vi "next chunk -- action stack.vi"(7 "stack action":T2, 8 "action list in":T1[](array[typedef]), 9 "next chunk action":T1=enum."init - uniform", 11 "command stack":T1[](array[typedef])) -> (1 "next chunk action out":T1=enum."init - uniform", 2 "stack is empty ?":bool, 3 "command stack out":T1[](array[typedef]))   [LabVIEW 2015]
uses:
  stack action -- control.ctl
  next chunk -- action.ctl
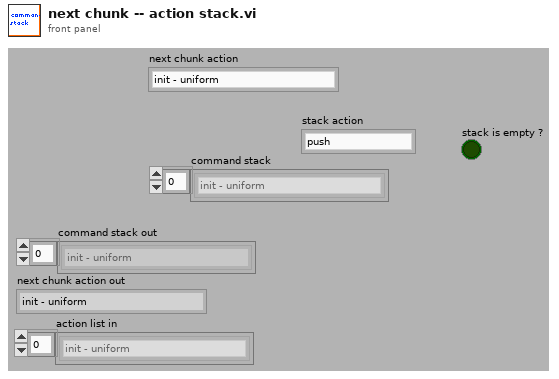
[diagram p1: front panel]
types:
  T1 = typedef "next chunk -- action.ctl" = enum16{"empty", "init - uniform", "next chunk - uniform", "next chunk - peaks are known", "init - peaks are known", ""}
  T2 = typedef "stack action -- control.ctl" = enum16{"push", "pop", "check", "init"}
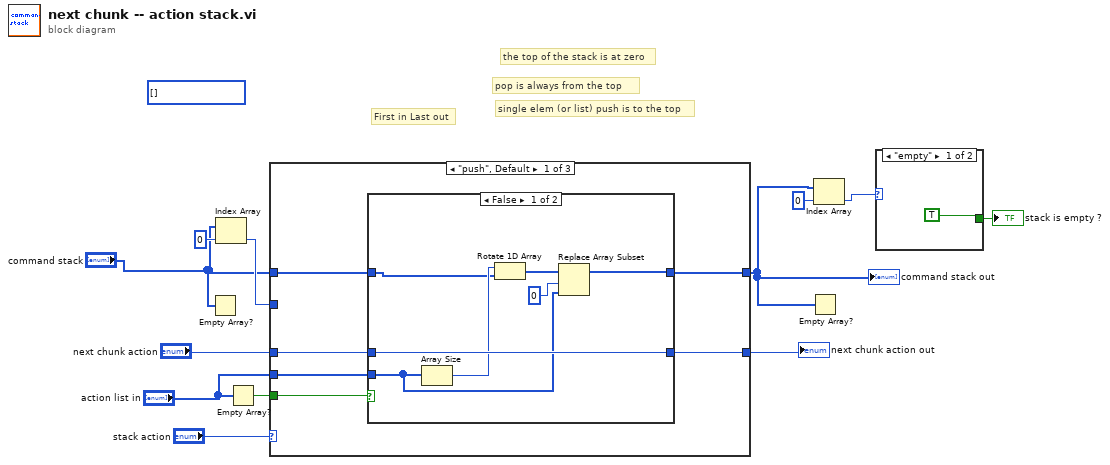
[diagram p0: block diagram]
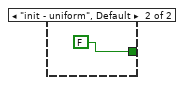
[diagram p2: hidden frame]
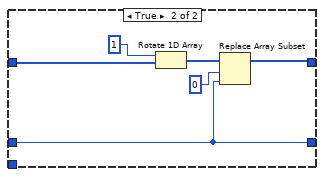
[diagram p3: hidden frame]
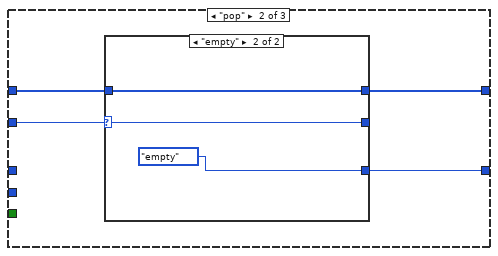
[diagram p4: hidden frame]
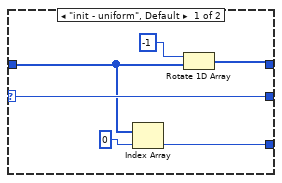
[diagram p5: hidden frame]
diagram:
  (unwired) T1[] [] items=["empty", "init - uniform", "next chunk - uniform", "next chunk - peaks are known", "init - peaks are known", ""] ("command stack")
  # "single elem (or list) push is to the top"
  # "pop is always from the top"
  # "First in Last out"
  # "the top of the stack is at zero"
  n1 = Empty Array?(array="command stack") -> ()  [unwired: 1 out]
  n2 = Index Array(array="command stack", index=0) -> (element=w9:T1)
  n3 = Empty Array?(array="action list in") -> (empty?=w11:bool)
  n4 = case shown="\"push\", Default" "stack action" {
    tunnel: [w18 w35 w45] -> w2
    tunnel: "command stack" -> [w17 w34 w45]
    tunnel: w9 -> [_ w33 _]
    tunnel: [w13 w32 w46] -> w3
    tunnel: "next chunk action" -> [w16 _ w46]
    tunnel: w11 -> [w15 _ _]
    tunnel: "action list in" -> [w14 _ _]
    frame "push", Default {
      n5 = case shown="False" w15 {
        tunnel: [w19 w26] -> w18
        tunnel: w17 -> [w23 w28]
        tunnel: w16 -> [w25 w29]
        tunnel: w14 -> [w20 _]
        tunnel: [w25 w29] -> w13
        frame False {
          n6 = Array Size(array=w20) -> (size(s)=w24:i32)
          n7 = Rotate 1D Array(1:w23, 2:w24) -> (0:w22:T1[])
          n8 = Replace Array Subset(array=w22, new element=w20, index=0) -> (w19:T1[])
        }
        frame True {
          n9 = Rotate 1D Array(1:w28, 2:1) -> (0:w31:T1[])
          n10 = Replace Array Subset(array=w31, new element=w29, index=0) -> (w26:T1[])
        }
      }
    }
    frame "pop" {
      n11 = case shown="\"empty\"" w33 {
        selector: w33 -> [w39 w43]
        tunnel: [w38 w44] -> w35
        tunnel: w34 -> [w36 w44]
        tunnel: [w40 next_chunk_--_action."empty" ("next chunk action")] -> w32
        tunnel: [w39 w43] -> _
        frame "init - uniform", Default {
          n12 = Index Array(array=w36, index=0) -> (element=w40:T1)
          n13 = Rotate 1D Array(1:w36, 2:-1) -> (0:w38:T1[])
        }
        frame "empty" {
        }
      }
    }
    frame "check" {
    }
  }
  "command stack out" <- w2
  "next chunk action out" <- w3
  n14 = Empty Array?(array=w2) -> ()  [unwired: 1 out]
  n15 = Index Array(array=w2, index=0) -> (element=w7:T1)
  n16 = case shown="\"empty\"" w7 {
    tunnel: [TRUE FALSE] -> w6
    frame "empty" {
    }
    frame "init - uniform", Default {
    }
  }
  "stack is empty ?" <- w6
